vi "GFITS_GetGeometryHeadersM.vi"(9 "readmode":string) -> (3 "Keywords out":string[][][](array[string]))   [LabVIEW 2016]
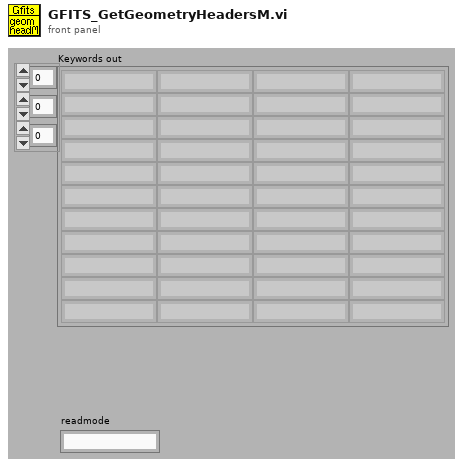
[diagram p1: front panel]
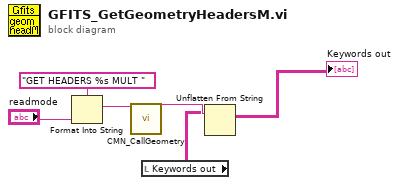
[diagram p0: block diagram]
diagram:
  n1 = Format Into String(format string="GET HEADERS %s MULT " ("Command"), "readmode") -> (resulting string=w5:string)  [unwired: 2 in, 1 out]
  n2 = call "CMN_CallGeometry.vi"("Command"=w5) -> ("ImmedReplyString"=w4:string)  [unwired: 1 in, 13 out]
  n3 = local read "Keywords out"() -> (w3:string[][][])
  n4 = Unflatten From String(type=w3, binary string=w4) -> (value=→"Keywords out":string[][][])  [unwired: 1 in, 4 out]
